vi "FEA_Model_Particle-Node_Converter.vi"(7 "mode":T1(ring), 8 "Node":i32, 9 "Nodes":i32[](array[numeric]), 10 "Particle":i32, 11 "Particles":i32[](array[numeric])) -> (0 "Particle":i32, 1 "Particles":i32[](array[numeric]), 2 "Node":i32, 3 "Nodes":i32[](array[numeric]))   [LabVIEW 2021, in "FEA_Model.lvclass"]
uses:
  FEA_Model.lvclass
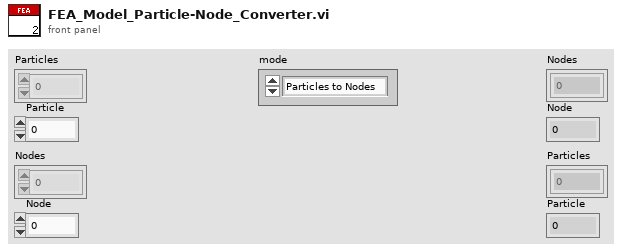
[diagram p1: front panel]
types:
  T1 = enum16{"Particles to Nodes", "Particle to Node", "Nodes to Particles", "Node to Particle"}
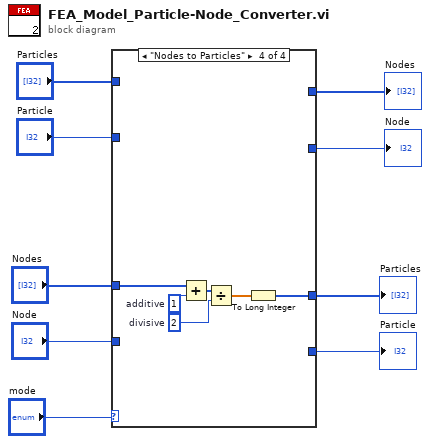
[diagram p0: block diagram]
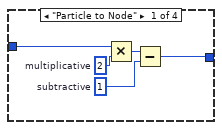
[diagram p2: hidden frame]
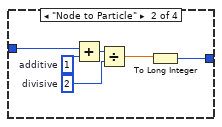
[diagram p3: hidden frame]
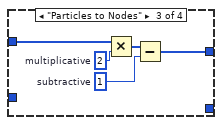
[diagram p4: hidden frame]
diagram:
  n1 = case shown="\"Nodes to Particles\"" "mode" {
    tunnel: "Particle" -> [w11 _ _ _]
    tunnel: "Particles" -> [_ _ w22 _]
    tunnel: [_ _ w21 _] -> w7
    tunnel: "Node" -> [_ w16 _ _]
    tunnel: "Nodes" -> [_ _ _ w27]
    tunnel: [_ w20 _ _] -> w4
    tunnel: [_ _ _ w31] -> w1
    tunnel: [w10 _ _ _] -> w2
    frame "Particle to Node" {
      w14 = 2  # multiplicative
      w12 = 1  # subtractive
      n2 = Multiply(x=w11, y=w14) -> (x*y=w13:i32)
      n3 = Subtract(x=w13, y=w12) -> (x-y=w10:i32)
    }
    frame "Node to Particle" {
      w19 = 2  # divisive
      w17 = 1  # additive
      n4 = Add(x=w16, y=w17) -> (x+y=w18:i32)
      n5 = Divide(x=w18, y=w19) -> (x/y=w15:dbl)
      n6 = To Long Integer(number=w15) -> (32bit integer=w20:i32)
    }
    frame "Particles to Nodes" {
      w25 = 2  # multiplicative
      w23 = 1  # subtractive
      n7 = Multiply(x=w22, y=w25) -> (x*y=w24:i32[])
      n8 = Subtract(x=w24, y=w23) -> (x-y=w21:i32[])
    }
    frame "Nodes to Particles" {
      w30 = 2  # divisive
      w28 = 1  # additive
      n9 = Add(x=w27, y=w28) -> (x+y=w29:i32[])
      n10 = Divide(x=w29, y=w30) -> (x/y=w26:dbl[])
      n11 = To Long Integer(number=w26) -> (32bit integer=w31:i32[])
    }
  }
  "Nodes" <- w7
  "Node" <- w2
  "Particles" <- w1
  "Particle" <- w4
